vi "TDMS_Location.vi"(4 "baseName":string="blah", 5 "basePath":path) -> (0 "location":path, 1 "filenname":string)   [LabVIEW 2021]
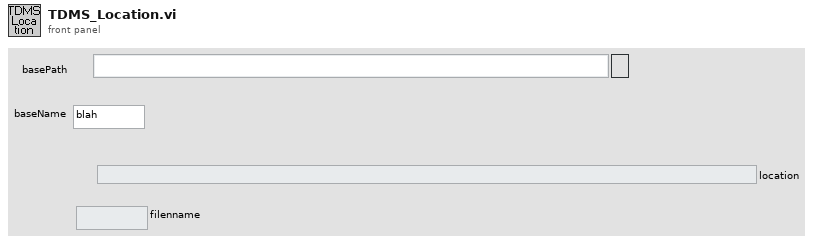
[diagram p1: front panel]
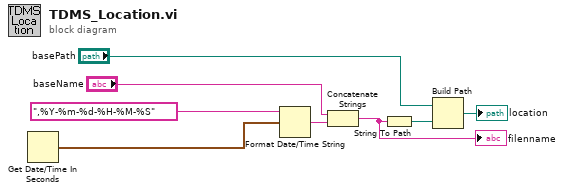
[diagram p0: block diagram]
diagram:
  n1 = Get Date/Time In Seconds() -> (seconds since 1Jan1904=w6:timestamp)
  n2 = Format Date/Time String(time format string (%c)=",%Y-%m-%d-%H-%M-%S", seconds (now)=w6) -> (date/time string=w7:string)  [unwired: 1 in]
  n3 = Concatenate Strings("baseName", w7) -> (w1:string)
  "filenname" <- w1
  n4 = String To Path(string=w1) -> (path=w3:path)
  n5 = Build Path(base path="basePath", name or relative path=w3) -> (appended path=→"location":path)
